vi "FireWriter.vi"() -> ()   [LabVIEW 2014]
doc: "This example demonstrates how to acquire a continuous amount of digital data based off of a sample clock.\n\nIt has been modified to save the resulting packed bits as a raw binary stream to disk."
uses:
  <vilib>/DAQmx/read.llb/DAQmx Read (Digital Wfm 1Chan NSamp).vi
  <vilib>/DAQmx/create/channels.llb/DAQmx Create Channel (DI-Digital Input).vi
  <vilib>/DAQmx/configure/timing.llb/DAQmx Timing (Sample Clock).vi
  <vilib>/DAQmx/configure/trigger.llb/DAQmx Start Trigger (Digital Edge).vi
  <vilib>/DAQmx/configure/trigger.llb/DAQmx Reference Trigger (Digital Edge).vi
  <vilib>/DAQmx/miscellaneous.llb/DAQmx Fill In Error Info.vi
  <vilib>/Waveform/DWDTOps.llb/DWDT Digital to Binary U8.vi
  <vilib>/DAQmx/create/channels.llb/DAQmx Create Channel (CO-Pulse Generation-Frequency).vi
  <vilib>/DAQmx/configure/timing.llb/DAQmx Timing (Implicit).vi
  <resource>/objmgr/daqmx.rc
panel:
  out "error out":errorcluster
  out "Status":string
  in  "fps":dbl=30.0 format="%0.2f"
  in  "file path (use dialog)":path=path "c:/data/fire3.dat"
  in  "Samples per Loop":i32=100000
  in  "Stop":bool
  out "Digital Waveform Graph":digitalwaveform(graph)
  in  "Sample Rate":dbl=100000.0
  out "Actual Sample Rate":dbl=1000.0 format="%0.2f"
  # "Ext. Trig. Settings"
  # "Acquired Data"
  # "Fire Record Settings"
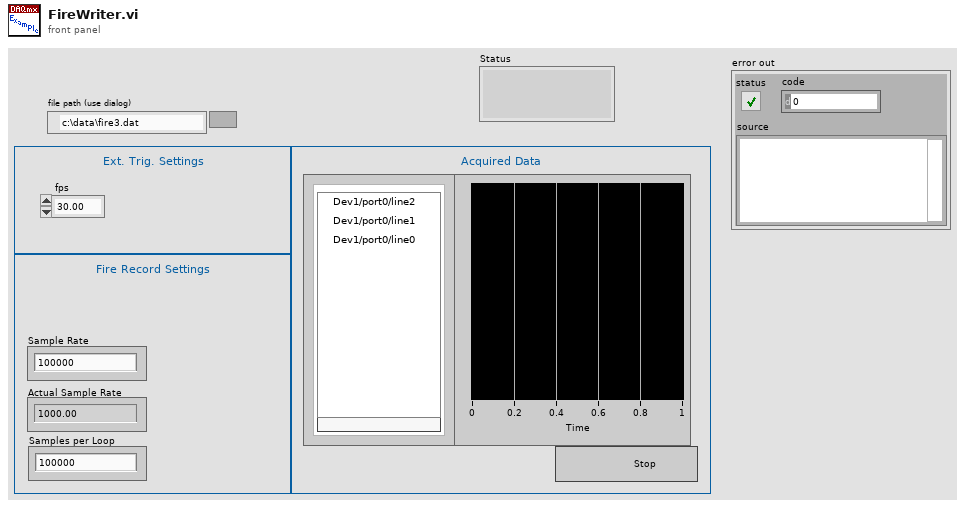
[diagram p1: front panel]
types:
  T1 = enum32{"No Trigger", "Digital Start", "Reference"}
  T2 = enum16{"big-endian, network order", "native, host order", "little-endian"}
  T3 = enum16{"open", "replace", "create", "open or create", "replace or create", "replace or create with confirmation"}
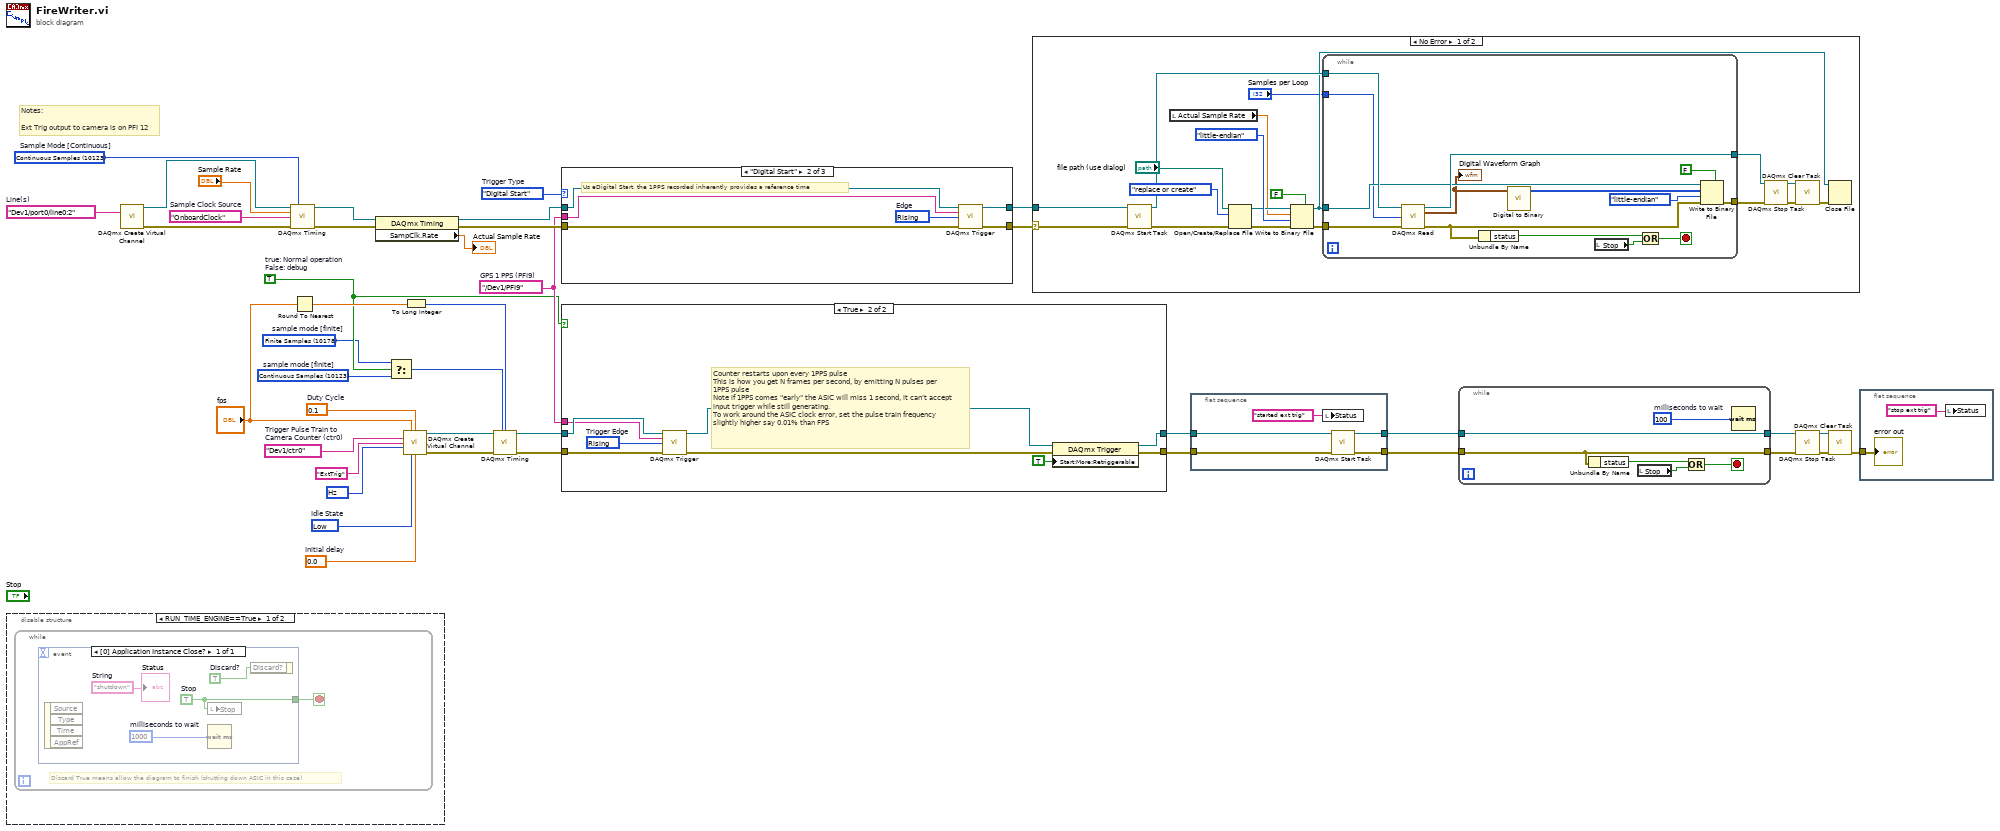
[diagram p0: block diagram]
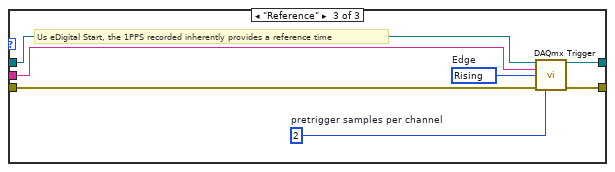
[diagram p6: hidden frame]
diagram:
  w3 = 10123 items=["Finite Samples"=10178, "Continuous Samples"=10123]  # sample mode [finite]
  w6 = TRUE  # true: Normal operation False: debug
  w33 = T1."Digital Start"  # Trigger Type
  w41 = tag "Dev1/port0/line0:2"  # Line(s)
  w39 = tag "OnboardClock"  # Sample Clock Source
  w11 = tag "/Dev1/PFI9"  # GPS 1 PPS (PFI9)
  w16 = tag "Dev1/ctr0"  # Trigger Pulse Train to  Camera Counter (ctr0)
  w19 = 10373 items=["Hz"=10373] ("units")
  w23 = 0.1  # Duty Cycle
  w24 = 0.0  # Initial delay
  w25 = 10214 items=["High"=10192, "Low"=10214]  # Idle State
  w2 = 10178 items=["Finite Samples"=10178, "Continuous Samples"=10123]  # sample mode [finite]
  w40 = 10123 items=["Finite Samples"=10178, "Continuous Samples"=10123, "Hardware Timed Single Point"=12522]  # Sample Mode [Continuous]
  # "Notes:\n\nExt Trig output to camera is on PFI 12"
  n1 = disable-structure shown="RUN_TIME_ENGINE==True" {
    frame condition #0 {
      n2 = while {
        stop <- w42 stop-if-true
        # "Discard True means allow the diagram to finish (shutting down ASIC in this case)"
        n3 = event shown="[0] Application Instance Close?" {
          selector: _ -> [_]
          dyn-events: _ -> [_]
          timeout: _ -> [_]
          tunnel: [w45] -> w42
          event Application Instance Close? {
            w43 = u32 1000  # milliseconds to wait
            w44 = "shutdown"  # String
            w46 = TRUE  # Discard?
            w45 = TRUE  # Stop
            n4 = event-data() -> ()  [unwired: 1 in, 4 out]
            n5 = local write "Stop"(w45) -> ()
            n6 = Wait (ms)(milliseconds to wait=w43) -> ()  [unwired: 1 out]
            n7 = event-data("Discard?"=w46) -> ()  [unwired: 1 in, 1 out]
            "Status" <- w44
          }
        }
      }
    }
    frame condition #1 (active) {
    }
  }
  n8 = call-poly <vilib>:"DAQmx Create Virtual Channel.vi"("lines"=w41) -> ("task out"=w37:refnum<k21>, "error out"=w36:errorcluster)  [unwired: 13 in]
  n9 = call-poly <vilib>:"DAQmx Timing.vi"("task/channels in"=w37, "sample mode"=w40, "rate"="Sample Rate", "source"=w39, "error in"=w36) -> ("task out"=w35:refnum<k21>, "error out"=w34:errorcluster)  [unwired: 9 in]
  n10 = Round To Nearest(number="fps") -> (nearest integer value=w17:dbl)
  n11 = property class="DAQmx Timing"(reference=w35, error in=w34) -> (reference out=w30:refnum<k21>, error out=w31:errorcluster, "SampClk.Rate"=→"Actual Sample Rate":dbl)
  n12 = Select(t=w2, s=w6, f=w3) -> (s? t:f=w4:i32)
  n13 = call-poly <vilib>:"DAQmx Create Virtual Channel.vi"("frequency"="fps", "duty cycle"=w23, "counter"=w16, "name to assign"="ExtTrig", "units"=w19, "idle state"=w25, "initial delay"=w24) -> ("task out"=w26:refnum<k21>, "error out"=w27:errorcluster)  [unwired: 7 in]
  n14 = To Long Integer(number=w17) -> (32bit integer=w5:i32)
  n15 = call-poly <vilib>:"DAQmx Timing.vi"("task/channels in"=w26, "sample mode"=w4, "samples per channel"=w5, "error in"=w27) -> ("task out"=w22:refnum<k21>, "error out"=w21:errorcluster)  [unwired: 10 in]
  n16 = case shown="\"Digital Start\"" w33 {
    tunnel: w30 -> [w48 w54 w61]
    tunnel: w31 -> [w47 w53 w60]
    tunnel: [w48 w52 w59] -> w32
    tunnel: [w47 w51 w58] -> w28
    tunnel: w11 -> [_ w49 w55]
    frame "No Trigger", Default {
    }
    frame "Digital Start" {
      w50 = 10280 items=["Rising"=10280, "Falling"=10171]  # Edge
      # "Us eDigital Start, the 1PPS recorded inherently provides a reference time"
      n17 = call-poly <vilib>:"DAQmx Trigger.vi"("task/channels in"=w54, "source"=w49, "edge"=w50, "error in"=w53) -> ("task out"=w52:refnum<k21>, "error out"=w51:errorcluster)  [unwired: 10 in]
    }
    frame "Reference" {
      w56 = u32 2  # pretrigger samples per channel
      w57 = 10280 items=["Rising"=10280, "Falling"=10171]  # Edge
      # "Us eDigital Start, the 1PPS recorded inherently provides a reference time"
      n18 = call-poly <vilib>:"DAQmx Trigger.vi"("task/channels in"=w61, "source"=w55, "edge"=w57, "error in"=w60, "pretrigger samples per channel"=w56) -> ("task out"=w59:refnum<k21>, "error out"=w58:errorcluster)  [unwired: 9 in]
    }
  }
  n19 = case shown="True" w6 {
    tunnel: w22 -> [w63 w72]
    tunnel: w21 -> [w62 w71]
    tunnel: [w63 w66] -> w15
    tunnel: [w62 w65] -> w14
    tunnel: w11 -> [_ w64]
    frame False {
    }
    frame True {
      w70 = 10280 items=["Rising"=10280, "Falling"=10171]  # Trigger Edge
      # "Counter restarts upon every 1PPS pulse\nThis is how you get N frames per second, by emitting N pulses per 1PPS pulse\nNote if 1PPS comes \"early\" the ASIC will miss 1 second, it can't accept input trigger while still generating.\nTo work around the ASIC clock error, set the pulse train frequency slightly higher say 0.01% than FPS"
      n20 = call-poly <vilib>:"DAQmx Trigger.vi"("task/channels in"=w72, "source"=w64, "edge"=w70, "error in"=w71) -> ("task out"=w68:refnum<k21>, "error out"=w67:errorcluster)  [unwired: 10 in]
      n21 = property class="DAQmx Trigger"(reference=w68, error in=w67, "Start:More:Retriggerable"=TRUE) -> (reference out=w66:refnum<k21>, error out=w65:errorcluster)
    }
  }
  n22 = case shown="No Error" w28 {
    selector: w28 -> [w75 _]
    tunnel: w32 -> [w91 _]
    frame No Error {
      n23 = call <vilib>:"DAQmx Start Task.vi"("task/channels in"=w91, "error in"=w75) -> ("task out"=w90:refnum<k21>, "error out"=w83:errorcluster)  [unwired: 12 in]
      n24 = local read "Actual Sample Rate"() -> (w74:dbl)
      n25 = Open/Create/Replace File(file path (use dialog)="file path (use dialog)", error in=w83, operation (0:open)=T3."replace or create") -> (refnum out=w77:refnum<file>, error out=w76:errorcluster)  [unwired: 3 in, 1 out]
      n26 = Write to Binary File(file (use dialog)=w77, data=w74, error in=w76, 5:FALSE ("prepend array or string size? (T)"), 9:T2."little-endian" ("byte order (0:big-endian, network order)")) -> (refnum out=w84:refnum<file>, error out=w82:errorcluster)  [unwired: 1 in, 1 out]
      n27 = while {
        tunnel: [w105] -> w87
        tunnel: [w96] -> w86
        tunnel: w82 -> [w104]
        tunnel: w90 -> [w103]
        tunnel: w84 -> [w99]
        tunnel: "Samples per Loop" -> [w92]
        stop <- w100 stop-if-true
        n28 = call-poly <vilib>:"DAQmx Read.vi"("task/channels in"=w103, "number of samples per channel"=w92, "error in"=w104) -> ("task out"=w105:refnum<k21>, "data"=w98:digitalwaveform, "error out"=w97:errorcluster)  [unwired: 10 in]
        "Digital Waveform Graph" <- w98
        n29 = Unbundle By Name(w97) -> ("status"=w102:bool)
        n30 = call-poly <vilib>:"Digital to Binary.vi"("digital waveform"=w98) -> ("binary array"=w95:u8[])  [unwired: 9 in, 1 out]
        n31 = local read "Stop"() -> (w101:bool)
        n32 = Or(x=w102, y=w101) -> (x .or. y?=w100:bool)
        n33 = Write to Binary File(file (use dialog)=w99, data=w95, error in=w97, 5:FALSE ("prepend array or string size? (T)"), 9:T2."little-endian" ("byte order (0:big-endian, network order)")) -> (error out=w96:errorcluster)  [unwired: 1 in, 2 out]
      }
      n34 = call <vilib>:"DAQmx Stop Task.vi"("task/channels in"=w87, "error in"=w86) -> ("task out"=w89:refnum<k21>, "error out"=w88:errorcluster)  [unwired: 12 in]
      n35 = call <vilib>:"DAQmx Clear Task.vi"("task in"=w89, "error in"=w88) -> ("error out"=w85:errorcluster)  [unwired: 13 in]
      n36 = Close File(refnum=w84, error in=w85) -> ()  [unwired: 2 out]
    }
    frame Error {
    }
  }
  n37 = flat-sequence {
    tunnel: w15 -> [w110]
    tunnel: w14 -> [w109]
    tunnel: [w108] -> w13
    tunnel: [w107] -> w12
    frame #0 {
      n38 = local write "Status"("started ext trig" ("String")) -> ()
      n39 = call <vilib>:"DAQmx Start Task.vi"("task/channels in"=w110, "error in"=w109) -> ("task out"=w108:refnum<k21>, "error out"=w107:errorcluster)  [unwired: 12 in]
    }
  }
  n40 = while {
    tunnel: w13 -> [w116]
    tunnel: [w116] -> w10
    tunnel: w12 -> [w112]
    tunnel: [w112] -> w8
    stop <- w113 stop-if-true
    w115 = u32 100  # milliseconds to wait
    n41 = Unbundle By Name(w112) -> ("status"=w111:bool)
    n42 = local read "Stop"() -> (w114:bool)
    n43 = Or(x=w111, y=w114) -> (x .or. y?=w113:bool)
    n44 = Wait (ms)(milliseconds to wait=w115) -> ()  [unwired: 1 out]
  }
  n45 = call <vilib>:"DAQmx Stop Task.vi"("task/channels in"=w10, "error in"=w8) -> ("task out"=w9:refnum<k21>, "error out"=w7:errorcluster)  [unwired: 12 in]
  n46 = call <vilib>:"DAQmx Clear Task.vi"("task in"=w9, "error in"=w7) -> ("error out"=w1:errorcluster)  [unwired: 13 in]
  n47 = flat-sequence {
    tunnel: w1 -> [w117]
    frame #0 {
      n48 = local write "Status"("stop ext trig" ("String")) -> ()
      "error out" <- w117
    }
  }
